vi "Update Shutter NP.vi"(8 "error in (no error)":errorcluster, 11 "Container in":refnum<class "Container.lvclass">) -> (0 "error out":errorcluster, 2 "Shutter-NP out":T1, 3 "Container out":refnum<class "Container.lvclass">)   [LabVIEW 2016]
uses:
  Classes/Shutter/Container/Container.lvclass
  Controls/Shutters.ctl
  Controls/Shutter Data.ctl
  Controls/Shutter States.ctl
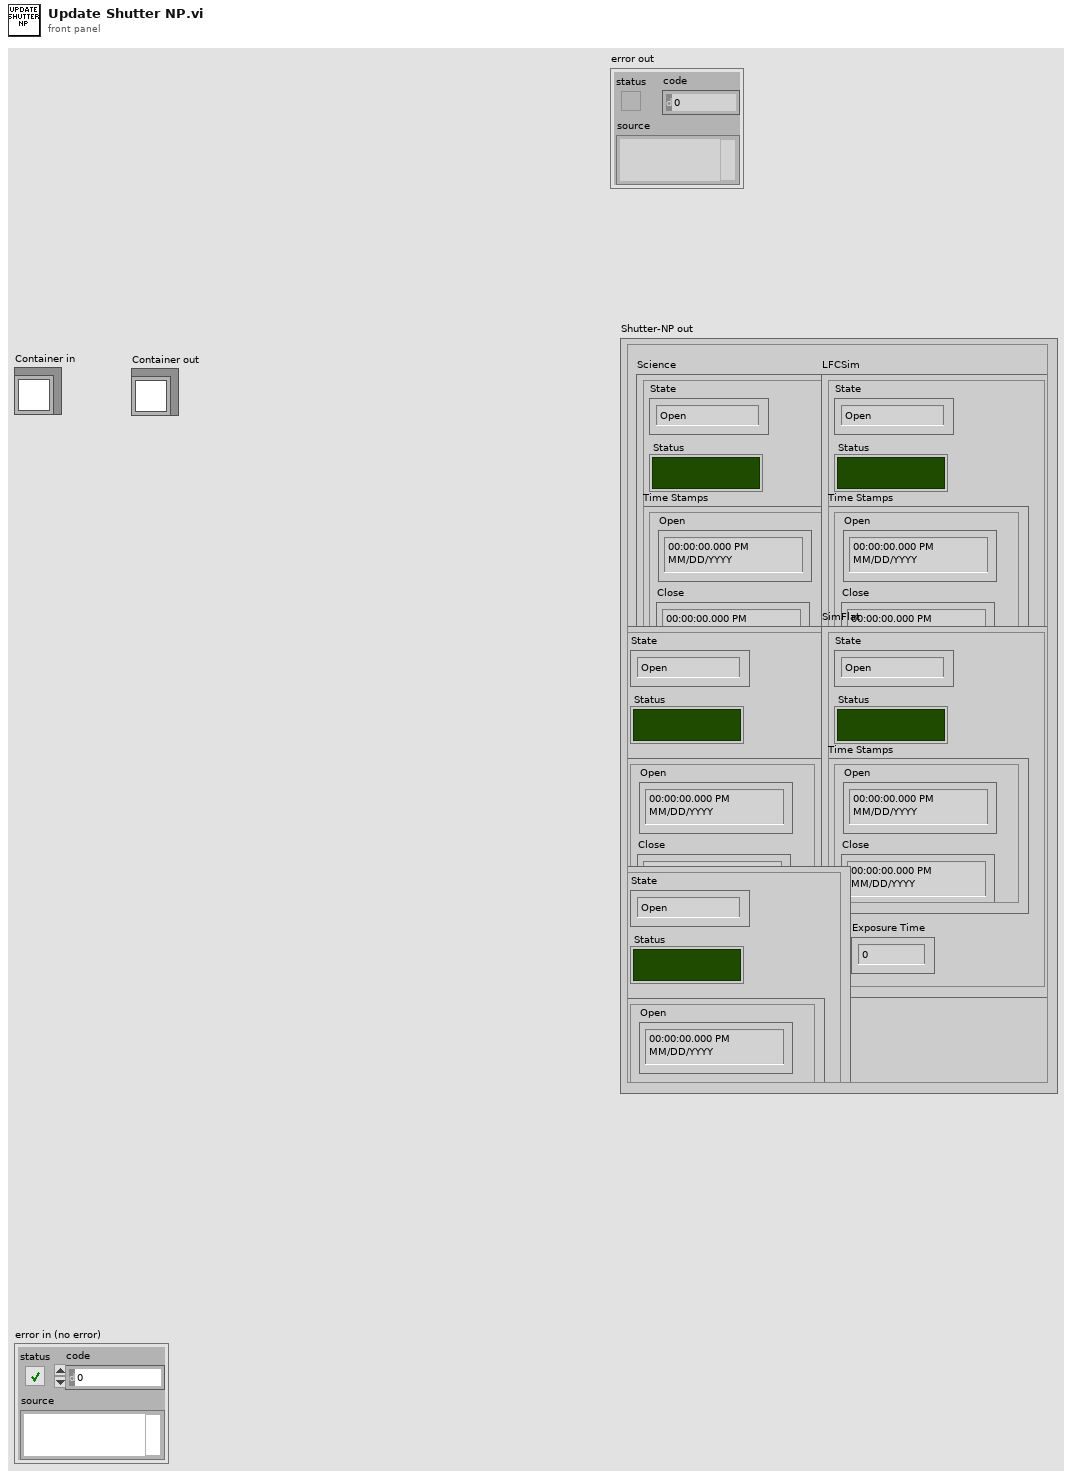
[diagram p1: front panel]
types:
  T1 = typedef "Shutters.ctl" = cluster{"Science":T2, "LFCSim":T2, "ExtendFlat":T2, "SimFlat":T2, "Solar":T2}
  T2 = typedef "Shutter Data.ctl" = cluster{"Status":bool, "State":T3, "Time Stamps":cluster{"Open":timestamp, "Close":timestamp}, "Exposure Time":dbl}
  T3 = typedef "Shutter States.ctl" = enum16{"Open", "Close", "Wait", "Off", "Arm", "Idle"}
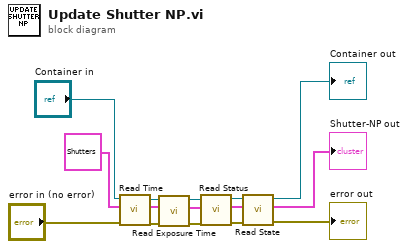
[diagram p0: block diagram]
diagram:
  n1 = call-dynamic "Read Time.vi"("error in (no error)"="error in (no error)", "Shutter-NP"=T1 {"Science"={"Status"=FALSE, "State"=enum."Open", "Time Stamps"={"Open"=timestamp(0 s since 1904-01-01), "Close"=timestamp(0 s since 1904-01-01)}, "Exposure Time"=0.0}, "LFCSim"={"Status"=FALSE, "State"=enum."Open", "Time Stamps"={"Open"=timestamp(0 s since 1904-01-01), "Close"=timestamp(0 s since 1904-01-01)}, "Exposure Time"=0.0}, "ExtendFlat"={"Status"=FALSE, "State"=enum."Open", "Time Stamps"={"Open"=timestamp(0 s since 1904-01-01), "Close"=timestamp(0 s since 1904-01-01)}, "Exposure Time"=0.0}, "SimFlat"={"Status"=FALSE, "State"=enum."Open", "Time Stamps"={"Open"=timestamp(0 s since 1904-01-01), "Close"=timestamp(0 s since 1904-01-01)}, "Exposure Time"=0.0}, "Solar"={"Status"=FALSE, "State"=enum."Open", "Time Stamps"={"Open"=timestamp(0 s since 1904-01-01), "Close"=timestamp(0 s since 1904-01-01)}, "Exposure Time"=0.0}}, "Container in"="Container in") -> ("error out"=w6:errorcluster, "Shutter-NP out"=w5:T1, "Container out"=w2:refnum<class "Container.lvclass">)  [unwired: 6 in]
  n2 = call-dynamic "Read Exposure Time.vi"("error in (no error)"=w6, "Shutter-NP In"=w5, "Container in"=w2) -> ("error out"=w1:errorcluster, "Shutter-NP Out"=w4:T1, "Container out"=w3:refnum<class "Container.lvclass">)  [unwired: 6 in]
  n3 = call-dynamic "Read Status.vi"("error in (no error)"=w1, "Shutter-NP"=w4, "Container in"=w3) -> ("error out"=w14:errorcluster, "Shutter-NP out"=w10:T1, "Container out"=w12:refnum<class "Container.lvclass">)  [unwired: 6 in]
  n4 = call-dynamic "Read State.vi"("error in (no error)"=w14, "Shutter-NP"=w10, "Container in"=w12) -> ("error out"=→"error out":errorcluster, "Shutter-NP out"=→"Shutter-NP out":T1, "Container out"=→"Container out":refnum<class "Container.lvclass">)  [unwired: 6 in]
